vi "Init Process.vi"(6 "Recipe State Data":refnum<data-value>, 8 "error in (no error)":errorcluster, 9 "Process State Data":refnum<data-value>, 10 "Interlock Q Class":refnum<class "Interlock Q Class.lvclass">, 11 "Recipe Controller in":refnum<class "Recipe Controller.lvclass">) -> (0 "error out":errorcluster, 3 "Recipe Controller out":refnum<class "Recipe Controller.lvclass">)   [LabVIEW 2022 SP3, in "Recipe Controller.lvclass"]
uses:
  Recipe Controller.lvclass
  XY Stage/Process Actor/Process Framework/Interlock Q Class/Interlock Q Class.lvclass
  XY Stage/Process Actor/Process Framework/Process State Data/Process State Data.lvclass
  Recipe Controller.lvclass/Recipe Controller.ctl
  Recipe State Data/Recipe State Data.lvclass
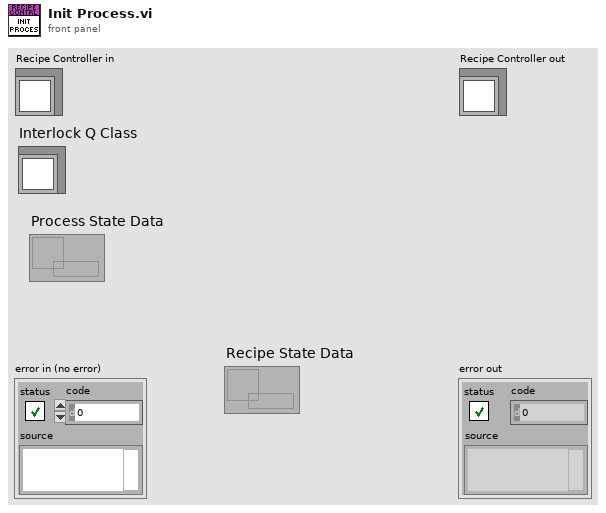
[diagram p1: front panel]
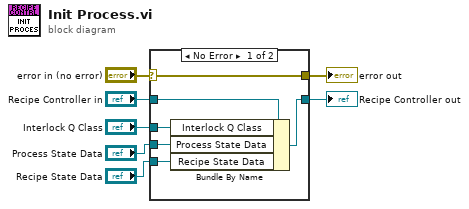
[diagram p0: block diagram]
diagram:
  n1 = case shown="No Error" "error in (no error)" {
    selector: "error in (no error)" -> [w12 w15]
    tunnel: [w12 w15] -> w6
    tunnel: [w11 w14] -> w4
    tunnel: "Recipe Controller in" -> [w13 w14]
    tunnel: "Interlock Q Class" -> [w10 _]
    tunnel: "Process State Data" -> [w9 _]
    tunnel: "Recipe State Data" -> [w8 _]
    frame No Error {
      n2 = Bundle By Name(cluster=w13, "Interlock Q Class"=w10, "Process State Data"=w9, "Recipe State Data"=w8) -> (w11:refnum<class "Recipe Controller.lvclass">)
    }
    frame Error {
    }
  }
  "error out" <- w6
  "Recipe Controller out" <- w4
